vi "generate radial profile.vi"(8 "error in (no error)":errorcluster caption="错误输入（无错误）", 9 "图像信号":dbl[][](array[numeric]), 10 "parameter for radial profile":T1={"R-step"=1.0, "R-min"=0.0, "R-max"=0.0, "num"=2, "x_center"=0.0, "y_center"=0.0, "校准起点"=0.0, "校准步长"=0.0, "校准终点"=0.0, "每步采样数（frame）"=0, "首尾去除帧数(frame)"=0, "Array R"=[], "Array profile"=[]}) -> (0 "error out":errorcluster caption="错误输出", 1 "ArrayR":sgl[](array[numeric]), 2 "profile":dbl[](array[numeric]))   [LabVIEW 2013]
doc: "该模板用于创建子VI。"
uses:
  parameter for radial profile.ctl
panel:
  in  "method":i32(ring)=3 items=["nearest", "bilinear", "bicubic", "bicubic spline"]
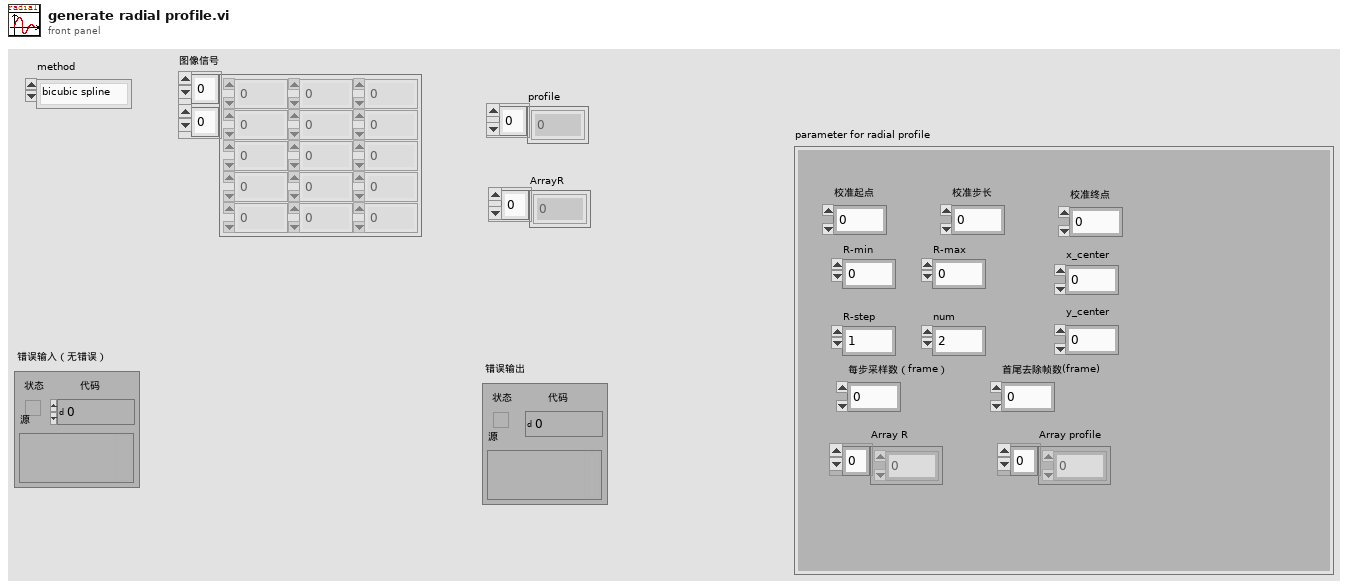
[diagram p1: front panel]
types:
  T1 = typedef "parameter for radial profile.ctl" = cluster{"R-step":sgl, "R-min":sgl, "R-max":sgl, "num":i32, "x_center":dbl, "y_center":dbl, "校准起点":dbl, "校准步长":dbl, "校准终点":dbl, "每步采样数（frame）":i32, "首尾去除帧数(frame)":i32, "Array R":dbl[], "Array profile":dbl[]}
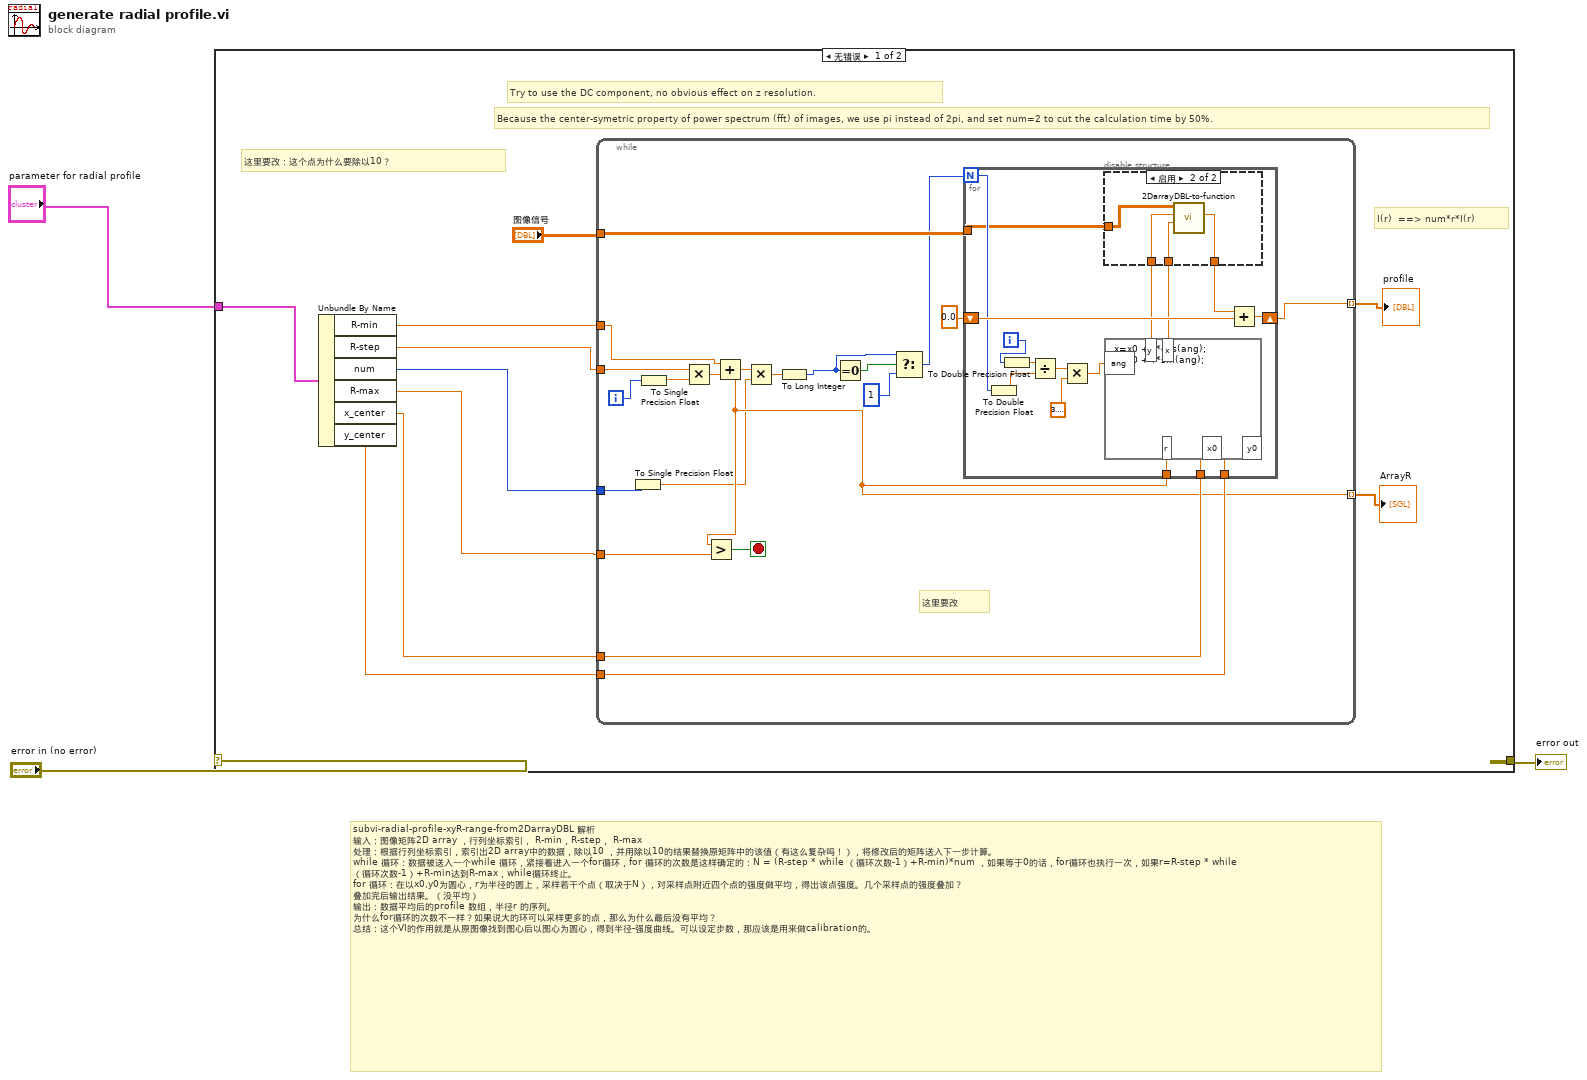
[diagram p0: block diagram]
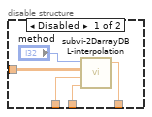
[diagram p2: hidden frame]
diagram:
  # "subvi-radial-profile-xyR-range-from2DarrayDBL 解析\n输入：图像矩阵2D array ，行列坐标索引， R-min，R-step， R-max\n处理：根据行列坐标索引，索引出2D array中的数据，除以10 ，并用除以10的结果替换原矩阵中的该值（有这么复杂吗！），将修改后的矩阵送入下一步计算。\nwhile 循环：数据被送入一个while 循环，紧接着进入一个for循环，for 循环的次数是这样确定的：N = (R-step * while （循环次数-1）+R-min)*num ，如果等于0的话，for循环也执行一次，如果r=R-step * while （循环次数-1）+R-min达到R-max，while循环终止。\nfor 循环：在以x0,y0为圆心，r为半径的圆上，采样若干个点（取决于N），对采样点附近四个点的强度做平均，得出该点强度。几个采样点的强度叠加？\n叠加完后输出结果。（没平均）\n输出：数据平均后的profile 数组，半径r 的序列。\n为什么for循环的次数不一样？如果说大的环可以采样更多的点，那么为什么最后没有平均？\n总结：这个VI的作用就是从原图像找到图心后以图心为圆心，得到半径-强度曲线。可以设定步数，那应该是用来做calibration的。"
  n1 = case shown="无错误" "error in (no error)" {
    selector: "error in (no error)" -> [_ w59]
    tunnel: [_ w59] -> w2
    tunnel: "parameter for radial profile" -> [w4 _]
    frame No Error {
      # "这里要改：这个点为什么要除以10？"
      # "Try to use the DC component, no obvious effect on z resolution."
      # "I(r)  ==> num*r*I(r)"
      # "Because the center-symetric property of power spectrum (fft) of images, we use pi instead of 2pi, and set num=2 to cut the calculation time by 50%."
      n2 = Unbundle By Name(w4) -> ("R-min"=w5:sgl, "R-step"=w6:sgl, "num"=w7:i32, "R-max"=w8:sgl, "x_center"=w10:dbl, "y_center"=w9:dbl)
      n3 = while {
        tunnel: "图像信号" -> [w33]
        tunnel: [w20] -> w13 mode=indexing
        tunnel: w9 -> [w31]
        tunnel: w10 -> [w30]
        tunnel: w6 -> [w26]
        tunnel: w5 -> [w29]
        tunnel: w8 -> [w24]
        tunnel: w7 -> [w23]
        tunnel: [w21] -> w12 mode=indexing
        i -> [w27]
        stop <- w25 stop-if-true
        # "这里要改"
        n4 = To Single Precision Float(number=w23) -> (single precision float=w14:sgl)
        n5 = To Single Precision Float(number=w27) -> (single precision float=w15:sgl)
        n6 = Multiply(x=w26, y=w15) -> (x*y=w28:sgl)
        n7 = Add(x=w29, y=w28) -> (x+y=w21:sgl)
        n8 = Greater?(x=w21, y=w24) -> (0:w25:bool)
        n9 = Multiply(x=w21, y=w14) -> (x*y=w22:sgl)
        n10 = To Long Integer(number=w22) -> (32bit integer=w18:i32)
        n11 = Equal To 0?(x=w18) -> (x = 0?=w19:bool)
        n12 = Select(t=w18, s=w19, f=1) -> (s? t:f=w16:i32)
        n13 = for {
          N: w16 -> [w42]
          tunnel: w33 -> [w39]
          tunnel: w30 -> [w49]
          tunnel: w31 -> [w48]
          shift-right: [w43] -> w20
          shift-left: 0.0 -> [w44]
          tunnel: w21 -> [w41]
          i -> [w47]
          n14 = To Double Precision Float(number=w42) -> (double precision float=w34:dbl)
          n15 = To Double Precision Float(number=w47) -> (double precision float=w35:dbl)
          n16 = Divide(x=w35, y=w34) -> (x/y=w46:dbl)
          n17 = Multiply(x=w46, y=3.141592653589793) -> (x*y=w45:dbl)
          n18 = formula code="x=x0 + r*cos(ang);\ny=y0 + r*sin(ang);"("x0"=w49, "y0"=w48, "ang"=w45, "r"=w41) -> ("x"=w37:dbl, "y"=w38:dbl)
          n19 = disable-structure shown="启用" {
            disable-tunnel: w39 -> [w54 w58]
            disable-tunnel: w38 -> [w53 w57]
            disable-tunnel: w37 -> [w52 w56]
            disable-tunnel: [w51 w55] -> w36
            frame Disabled {
              n20 = call "subvi-2DarrayDBL-interpolation.vi"("xi"=w52, "yi"=w53, "2D array"=w54, "method"="method") -> ("f(x,y)"=w51:dbl)  [unwired: 2 out]
            }
            frame Enabled {
              n21 = call "2DarrayDBL-to-function.vi"("X"=w56, "Y"=w57, "2D array"=w58) -> ("f(x,y)"=w55:dbl)  [unwired: 6 in, 2 out]
            }
          }
          n22 = Add(x=w36, y=w44) -> (x+y=w43:dbl)
        }
      }
      "profile" <- w13
      "ArrayR" <- w12
    }
    frame Error {
    }
  }
  "error out" <- w2
